vi "newsubvi Robot GoTo Focus.vi"(2 "Magnification":u8, 3 "Objective":u8, 4 "VISA In":refnum<visa-resource-name>) -> (0 "error out":errorcluster, 1 "VISA Out":refnum<visa-resource-name>)   [LabVIEW 2012]
uses:
  <vilib>/Utility/config.llb/Read Key (I32).vi
  <vilib>/Utility/config.llb/NI_LVConfig.lvlib
panel:
  out "Target":i32
  out "Feedback":i32
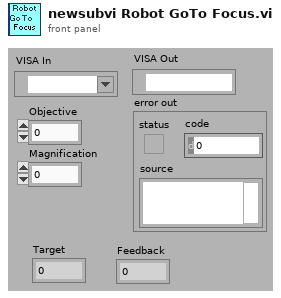
[diagram p1: front panel]
types:
  T1 = enum16{"Undefined", "Focus", "XMin", "YMax", "XY"}
  T2 = typedef "NI_LVConfig.lvlib/Config Data RefNum.ctl" = refnum<k1>
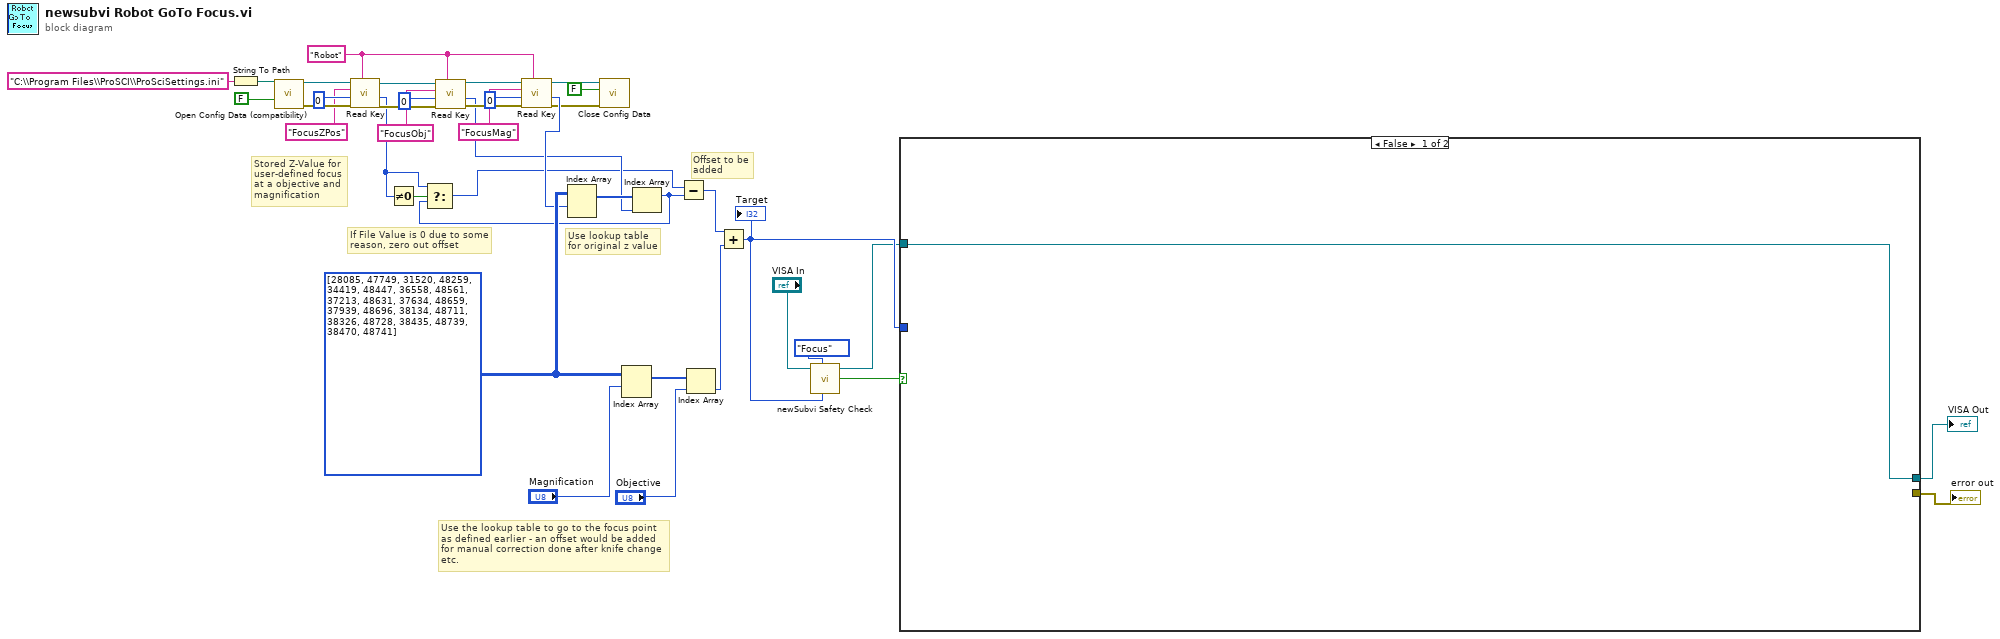
[diagram p0: block diagram]
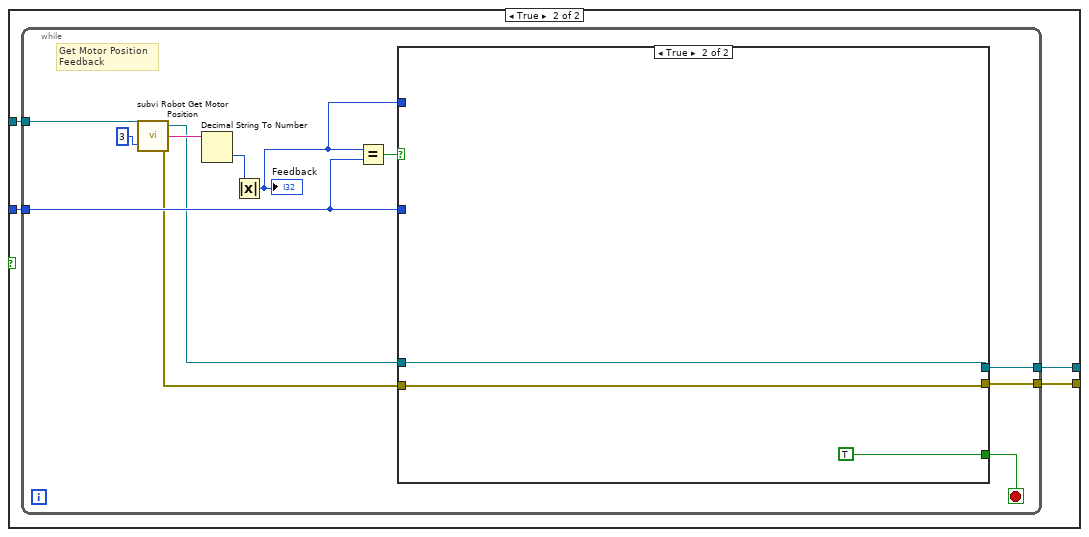
[diagram p2: hidden frame]
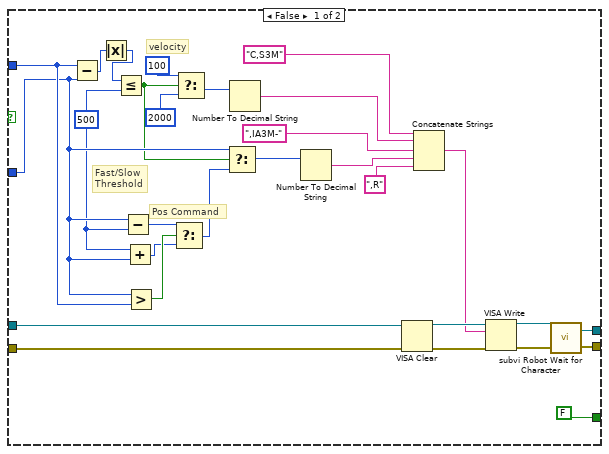
[diagram p3: hidden frame]
diagram:
  w21 = "Robot" ("section")
  w19 = i32[][] [[28085, 47749], [31520, 48259], [34419, 48447], [36558, 48561], [37213, 48631], [37634, 48659], [37939, 48696], [38134, 48711], [38326, 48728], [38435, 48739], [38470, 48741]] ("array")
  # "If File Value is 0 due to some\nreason, zero out offset"
  # "Offset to be\nadded"
  # "Stored Z-Value for\nuser-defined focus\nat a objective and\nmagnification"
  # "Use lookup table\nfor original z value"
  # "Use the lookup table to go to the focus point\nas defined earlier - an offset would be added\nfor manual correction done after knife change\netc."
  n1 = String To Path(string="C:\\Program Files\\ProSCI\\ProSciSettings.ini") -> (path=w35:path)
  n2 = call <vilib>:"Open Config Data (compatibility).vi"("create file if necessary (T)"=FALSE ("create file if necessary? (T)"), "configuration file path"=w35) -> ("error out"=w31:errorcluster, "refnum"=w33:T2)  [unwired: 7 in, 1 out]
  n3 = call-poly <vilib>:"Read Key.vi"("section"=w21, "error in (no error)"=w31, "default value"=0, "key"="FocusZPos", "refnum"=w33) -> ("error out"=w24:errorcluster, "value"=w9:i32, "refnum out"=w25:T2)  [unwired: 4 out]
  n4 = Not Equal To 0?(x=w9) -> (x != 0?=w11:bool)
  n5 = call-poly <vilib>:"Read Key.vi"("section"=w21, "error in (no error)"=w24, "default value"=0, "key"="FocusObj", "refnum"=w25) -> ("error out"=w22:errorcluster, "value"=w17:i32, "refnum out"=w23:T2)  [unwired: 4 out]
  n6 = call-poly <vilib>:"Read Key.vi"("section"=w21, "error in (no error)"=w22, "default value"=0, "key"="FocusMag", "refnum"=w23) -> ("error out"=w12:errorcluster, "value"=w18:i32, "refnum out"=w13:T2)  [unwired: 4 out]
  n7 = Index Array(array=w19, index (row)=w18) -> (element=w20:i32[])  [unwired: 1 in]
  n8 = call <vilib>:"Close Config Data.vi"("error in (no error)"=w12, "write file if changed (T)"=FALSE ("write configuration file? (T)"), "refnum"=w13) -> ()  [unwired: 9 out]
  n9 = Index Array(array=w19, index (row)="Magnification") -> (element=w38:i32[])  [unwired: 1 in]
  n10 = Index Array(array=w20, index=w17) -> (element=w8:i32)
  n11 = Select(t=w9, s=w11, f=w8) -> (s? t:f=w10:i32)
  n12 = Subtract(x=w10, y=w8) -> (x-y=w16:i32)
  n13 = Index Array(array=w38, index="Objective") -> (element=w15:i32)
  n14 = Add(x=w16, y=w15) -> (x+y=w6:i32)
  "Target" <- w6
  n15 = call "newSubvi Safety Check.vi"("VISA In"="VISA In", "SafetyCheck"=T1."Focus", "ZTarget"=w6) -> ("VISA Out"=w3:refnum<visa-resource-name>, "Safe"=w5:bool)  [unwired: 2 in, 1 out]
  n16 = case shown="False" w5 {
    tunnel: w6 -> [_ w44]
    tunnel: w3 -> [w40 w43]
    tunnel: [w40 w42] -> w2
    tunnel: [_ w41] -> w1
    frame False {
    }
    frame True {
      n17 = while {
        tunnel: w44 -> [w51]
        tunnel: w43 -> [w49]
        tunnel: [w46] -> w42
        tunnel: [w45] -> w41
        stop <- w53 stop-if-true
        # "Get Motor Position\nFeedback"
        n18 = call "subvi Robot Get Motor Position.vi"("VISA In"=w49, "Motor Number"=3) -> ("VISA Out"=w47:refnum<visa-resource-name>, "Motor Position"=w56:string, "error out"=w48:errorcluster)  [unwired: 1 out]
        n19 = Decimal String To Number(string=w56) -> (number=w55:i32)  [unwired: 3 out]
        n20 = Absolute Value(x=w55) -> (abs(x)=w52:i32)
        "Feedback" <- w52
        n21 = Equal?(x=w52, y=w51) -> (x = y?=w54:bool)
        n22 = case shown="True" w54 {
          tunnel: [FALSE TRUE] -> w53
          tunnel: w52 -> [w85 _]
          tunnel: w51 -> [w84 _]
          tunnel: w48 -> [w82 w86]
          tunnel: w47 -> [w81 w87]
          tunnel: [w58 w87] -> w46
          tunnel: [w57 w86] -> w45
          frame False {
            w76 = 500 ("y")
            # "Fast/Slow\nThreshold"
            # "Pos Command"
            # "velocity"
            n23 = Subtract(x=w85, y=w84) -> (x-y=w65:i32)
            n24 = Absolute Value(x=w65) -> (abs(x)=w64:i32)
            n25 = Less Or Equal?(x=w64, y=w76) -> (x <= y?=w68:bool)
            n26 = Subtract(x=w84, y=w76) -> (x-y=w77:i32)
            n27 = Add(x=w76, y=w84) -> (x+y=w75:i32)
            n28 = Greater?(x=w84, y=w85) -> (0:w78:bool)
            n29 = Select(t=w77, s=w78, f=w75) -> (s? t:f=w66:i32)
            n30 = Select(t=100 ("y"), s=w68, f=2000 ("y")) -> (s? t:f=w74:i32)
            n31 = Select(t=w84, s=w68, f=w66) -> (s? t:f=w67:i32)
            n32 = Number To Decimal String(number=w74) -> (decimal integer string=w70:string)  [unwired: 1 out]
            n33 = Number To Decimal String(number=w67) -> (decimal integer string=w73:string)  [unwired: 1 out]
            n34 = VISA Clear(VISA resource name=w81, error in (no error)=w82) -> (VISA resource name out=w63:refnum<visa-resource-name>, error out=w62:errorcluster)
            n35 = Concatenate Strings("C,S3M", w70, ",IA3M-", w73, ",R" ("Text to Send")) -> (w59:string)
            n36 = VISA Write(VISA resource name=w63, write buffer=w59, error in (no error)=w62) -> (VISA resource name out=w61:refnum<visa-resource-name>, error out=w60:errorcluster)  [unwired: 1 out]
            n37 = call "subvi Robot Wait for Character.vi"("error in"=w60, "VISA In"=w61) -> ("error out"=w57:errorcluster, "VISA Out"=w58:refnum<visa-resource-name>)
          }
          frame True {
          }
        }
      }
    }
  }
  "VISA Out" <- w2
  "error out" <- w1
